vi "magnetic-field.vi"(3 "dist to goal nullify":dbl=200.0, 5 "max angle (greater)":dbl=1.1 format="%#_13g", 6 "max force":dbl=3.0 format="%#_13g", 7 "obstacle influence radius":dbl=700.0 format="%#_13g", 8 "goal pos":dbl[](array[numeric])=[0.0, 0.0] format="%#_13g", 9 "obstacle pos":dbl[](array[numeric])=[0.0, 1e-10] format="%#_13g", 11 "robot pos":dbl[](array[numeric])=[0.0, 0.0] format="%#_13g") -> (2 "magnetic force":dbl[](array[numeric]))   [LabVIEW 2020]
uses:
  <vilib>/Analysis/_algsub.llb/Vector Norm Type.ctl
  <vilib>/Analysis/baseanly.llb/Unit Vector (DBL).vi
  <vilib>/Analysis/coordinate.llb/2D Cartesian Coordinate Rotation (Scalar).vi
  <vilib>/Analysis/baseanly.llb/Real Dot Product.vi
  <vilib>/Analysis/NI_AALBase.lvlib
  <vilib>/Analysis/NI_AALPro.lvlib
panel:
  in  "too close":dbl=90.0 format="%#_13g"
  in  "y wrap around switch eps":dbl=20.0 format="%#_13g"
  out "magnitude":dbl
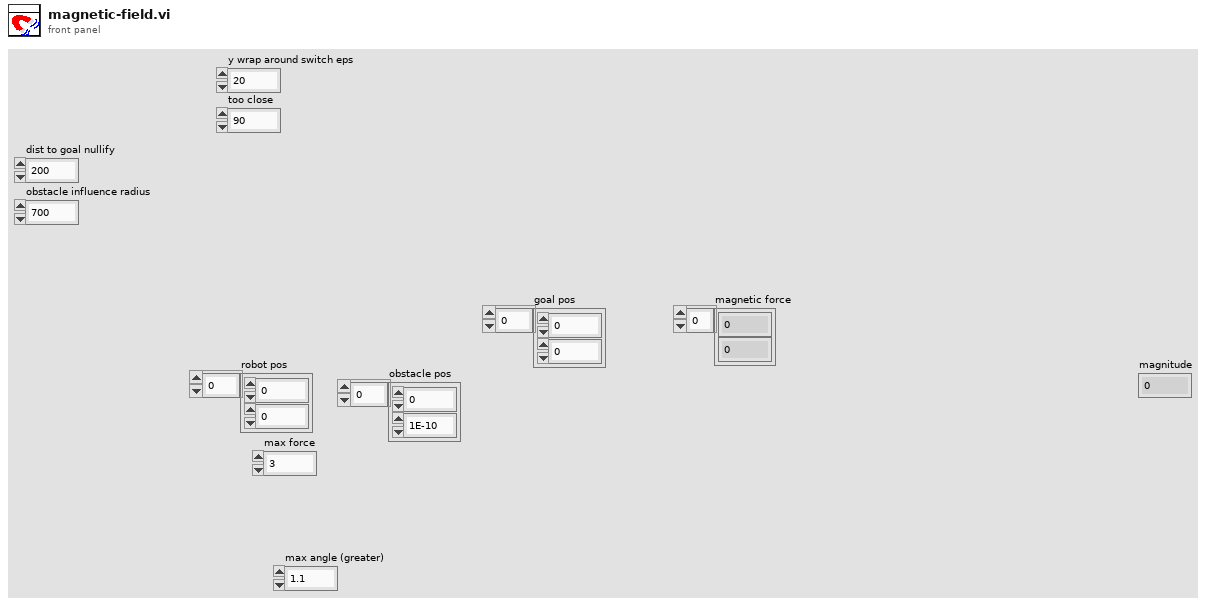
[diagram p1: front panel]
types:
  T1 = typedef "NI_AALPro.lvlib/Vector Norm Type.ctl" = u16
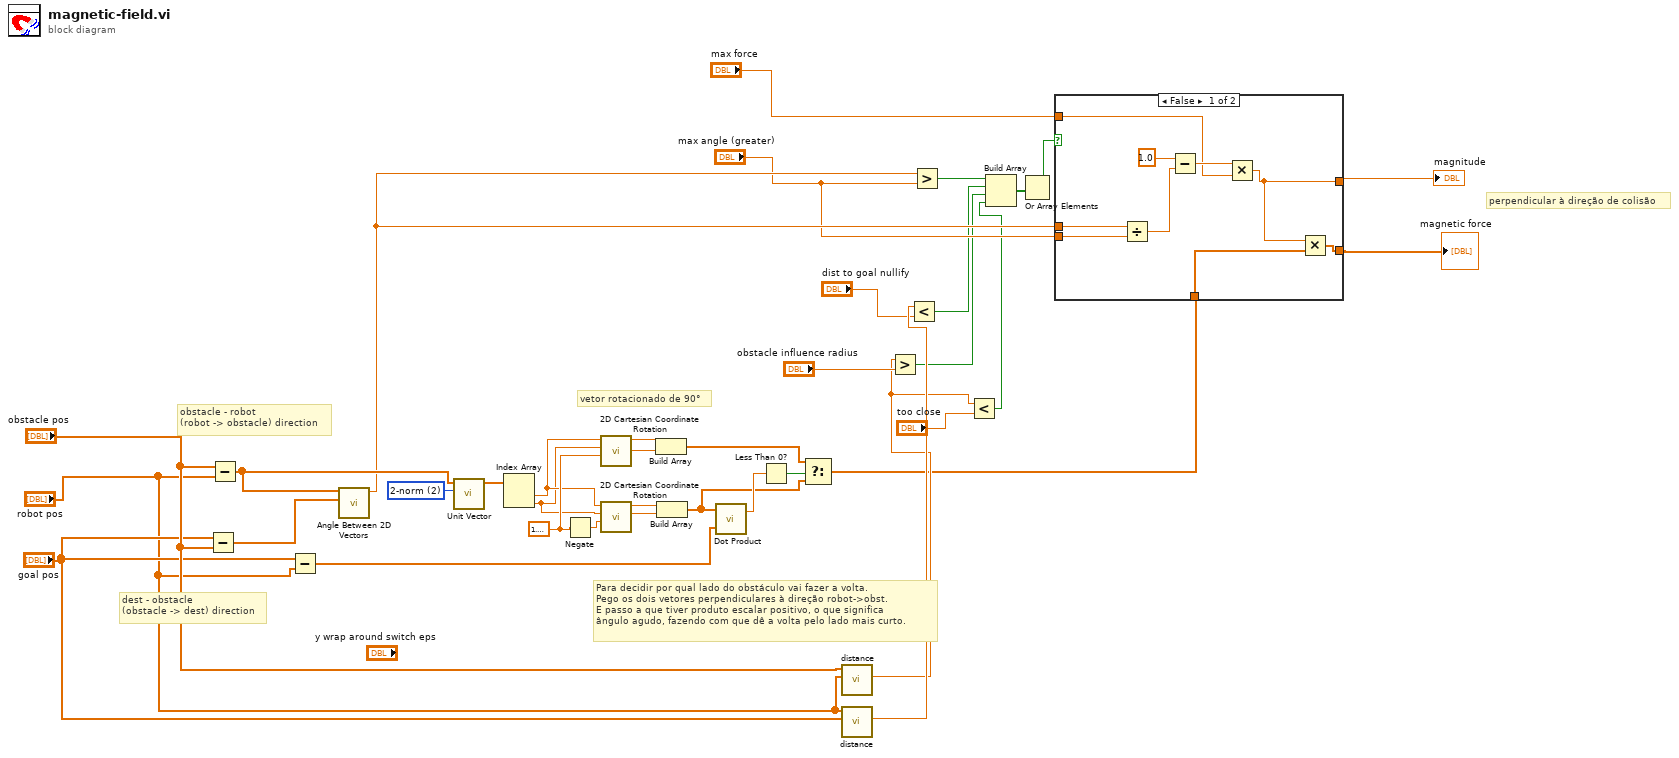
[diagram p0: block diagram]
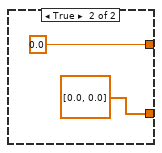
[diagram p2: hidden frame]
diagram:
  w16 = 1.5707963267948966
  w34 = T1 2 items=["1-norm"=1, "2-norm"=2, "Inf-norm"=3, "-Inf-norm"=4, "User Defined"=5] ("norm type")
  # "Para decidir por qual lado do obstáculo vai fazer a volta.\nPego os dois vetores perpendiculares à direção robot->obst.\nE passo a que tiver produto escalar positivo, o que significa\nângulo agudo, fazendo com que dê a volta pelo lado mais curto."
  # "perpendicular à direção de colisão"
  # "vetor rotacionado de 90°"
  # "obstacle - robot\n(robot -> obstacle) direction"
  # "dest - obstacle\n(obstacle -> dest) direction"
  n1 = Subtract(x="goal pos", y="obstacle pos") -> (x-y=w36:dbl[])
  n2 = Subtract(x="obstacle pos", y="robot pos") -> (x-y=w35:dbl[])
  n3 = Subtract(x="goal pos", y="robot pos") -> (x-y=w6:dbl[])
  n4 = call "Angle Between 2D Vectors.vi"("Array"=w36, "Array 2"=w35) -> ("angleBetweenVectors"=w33:dbl)  [unwired: 9 in]
  n5 = call-poly <vilib>:"Unit Vector.vi"("norm type"=w34, "Input Vector"=w35) -> ("Unit Vector"=w17:dbl[])  [unwired: 7 in, 2 out]
  n6 = Index Array(array=w17) -> (element #1=w14:dbl, element #2=w13:dbl)  [unwired: 2 in]
  n7 = Negate(x=w16) -> (-x=w15:dbl)
  n8 = call-poly <vilib>:"2D Cartesian Coordinate Rotation.vi"("theta"=w16, "y"=w13, "x"=w14) -> ("y out"=w11:dbl, "x out"=w12:dbl)  [unwired: 6 in, 1 out]
  n9 = call-poly <vilib>:"2D Cartesian Coordinate Rotation.vi"("theta"=w15, "y"=w13, "x"=w14) -> ("y out"=w9:dbl, "x out"=w10:dbl)  [unwired: 6 in, 1 out]
  n10 = Build Array(w12, w11) -> (w3:dbl[])
  n11 = Build Array(w10, w9) -> (w2:dbl[])
  n12 = call-poly <vilib>:"Dot Product.vi"("Y Vector"=w6, "X Vector"=w2) -> ("X * Y"=w4:dbl)  [unwired: 1 out]
  n13 = Less Than 0?(x=w4) -> (x < 0?=w5:bool)
  n14 = Select(t=w3, s=w5, f=w2) -> (s? t:f=w1:dbl[])
  n15 = call "distance.vi"("P1"="robot pos", "P2"="obstacle pos") -> ("Dist P1P2"=w21:dbl)  [unwired: 9 in]
  n16 = call "distance.vi"("P1"="goal pos", "P2"="robot pos") -> ("Dist P1P2"=w30:dbl)  [unwired: 9 in]
  n17 = Greater?(x=w21, y="obstacle influence radius") -> (0:w24:bool)
  n18 = Less?(x=w30, y="dist to goal nullify") -> (x < y?=w25:bool)
  n19 = Greater?(x=w33, y="max angle (greater)") -> (0:w26:bool)
  n20 = Less?(x=w21, y="too close") -> (x < y?=w19:bool)
  n21 = Build Array(w26, w25, w24, w19) -> (w23:bool[])
  n22 = Or Array Elements(Boolean array=w23) -> (logical OR=w22:bool)
  n23 = case shown="False" w22 {
    tunnel: [w39 0.0] -> w37
    tunnel: w33 -> [w46 _]
    tunnel: "max angle (greater)" -> [w44 _]
    tunnel: "max force" -> [w41 _]
    tunnel: w1 -> [w40 _]
    tunnel: [w38 dbl[] [0.0, 0.0]] -> w18
    frame False {
      n24 = Divide(x=w46, y=w44) -> (x/y=w43:dbl)
      n25 = Subtract(x=1.0, y=w43) -> (x-y=w42:dbl)
      n26 = Multiply(x=w42, y=w41) -> (x*y=w39:dbl)
      n27 = Multiply(x=w39, y=w40) -> (x*y=w38:dbl[])
    }
    frame True {
    }
  }
  "magnitude" <- w37
  "magnetic force" <- w18
